vi "Initialize.vi"(8 "error in (no error)":errorcluster, 11 "VISA resource name":refnum<visa-resource-name>) -> (0 "error out":errorcluster, 3 "VISA resource name out":refnum<visa-resource-name>)   [LabVIEW 2023, in "Marlin Instrument Driver.lvlib"]
doc: "Establishes communication with the instrument and optionally performs an instrument identification query and/or an instrument reset. It also places the instrument in a default state needed for other instrument driver operations. Therefore, call this VI before calling other instrument driver VIs for this instrument. Generally, you need to call the <b>Initialize</b> VI only once at the beginning of an application."
uses:
  Marlin Instrument Driver.lvlib
panel:
  # "(c) 2021 Proper Printing.  ALL RIGHTS RESERVED."
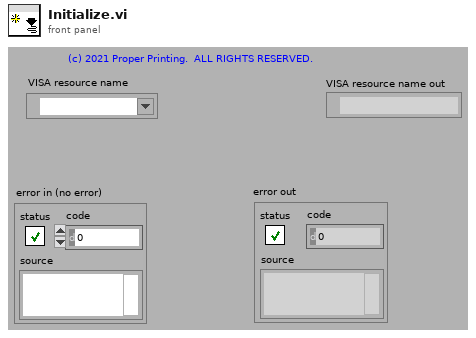
[diagram p1: front panel]
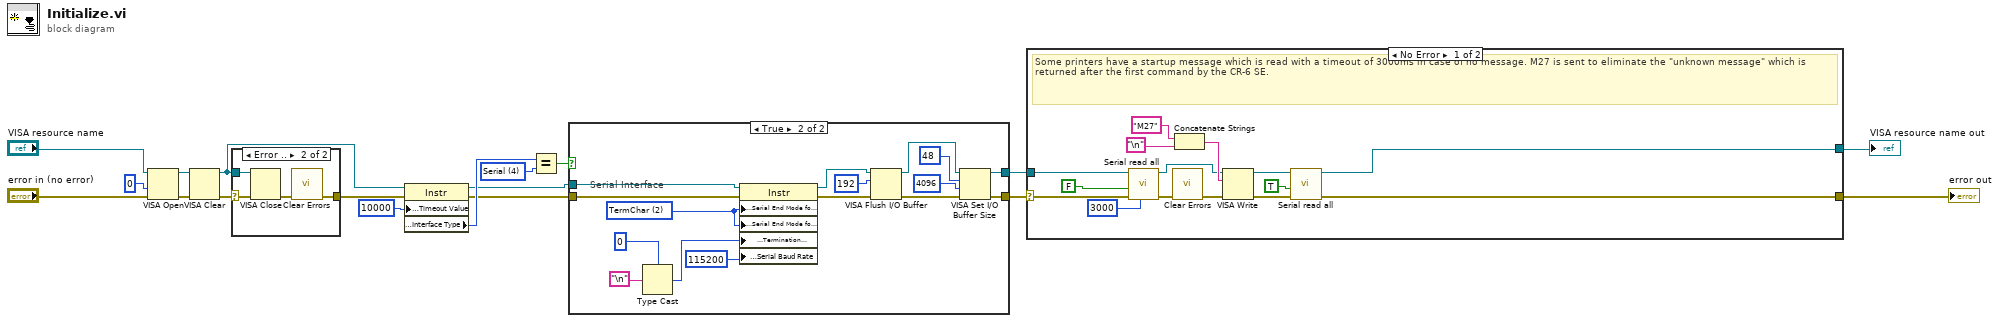
[diagram p0: block diagram]
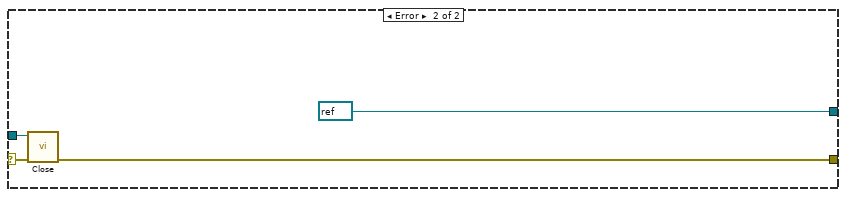
[diagram p4: hidden frame]
diagram:
  w11 = u16 4 items=["GPIB"=1, "VXI"=2, "GPIB-VXI"=3, "Serial"=4, "PXI"=5, "TCPIP"=6, "USB"=7] ("Interface Information:Interface Type")
  n1 = VISA Open(access mode=u32 0, error in (no error)="error in (no error)", VISA resource name="VISA resource name") -> (VISA resource name=w9:refnum<visa-resource-name>, error out=w8:errorcluster)  [unwired: 2 in]
  n2 = VISA Clear(VISA resource name=w9, error in (no error)=w8) -> (VISA resource name out=w1:refnum<visa-resource-name>, error out=w3:errorcluster)
  n3 = case shown="Error .." w3 {
    selector: w3 -> [w19 w22]
    tunnel: w1 -> [_ w23]
    tunnel: [w19 w20] -> w2
    frame No Error {
    }
    frame Error {
      n4 = VISA Close(VISA resource name=w23, error in (no error)=w22) -> (error out=w21:errorcluster)
      n5 = call <vilib>:"Clear Errors.vi"("error in (no error)"=w21) -> ("error out"=w20:errorcluster)  [unwired: 5 in, 1 out]
    }
  }
  n6 = property class="Instr"(reference=w1, error in=w2, "General Settings:Timeout Value"=u32 10000) -> (reference out=w14:refnum<visa-resource-name>, error out=w13:errorcluster, "Interface Information:Interface Type"=w16:u16)
  n7 = Equal?(x=w16, y=w11) -> (x = y?=w12:bool)
  n8 = case shown="True" w12 {
    tunnel: [w24 w38] -> w5
    tunnel: [w25 w35] -> w4
    tunnel: w14 -> [w24 w40]
    tunnel: w13 -> [w25 w41]
    frame False {
      # "GPIB, TCP/IP, and USB Interface"
    }
    frame True {
      w28 = u16 2 items=["None", "LastBit", "TermChar"] ("Serial Settings:Serial End Mode for Reads")
      # "Serial Interface"
      n9 = Type Cast(type=u8 0, x="\n" ("Line Feed Constant")) -> (*(type *) &x=w27:u8)
      n10 = property class="Instr"(reference=w40, error in=w41, "Serial Settings:Serial End Mode for Reads"=w28, "Serial Settings:Serial End Mode for Writes"=w28, "Message Based Settings:Termination Character"=w27, "Serial Settings:Serial Baud Rate"=u32 115200 ("Serial Settings:Baud Rate")) -> (reference out=w34:refnum<visa-resource-name>, error out=w37:errorcluster)
      n11 = VISA Flush I/O Buffer(VISA resource name=w34, mask (16)=u16 192, error in (no error)=w37) -> (VISA resource name out=w39:refnum<visa-resource-name>, error out=w36:errorcluster)
      n12 = VISA Set I/O Buffer Size(VISA resource name=w39, mask (16)=u16 48, size (4096)=u32 4096 ("size (0)"), error in (no error)=w36) -> (VISA resource name out=w38:refnum<visa-resource-name>, error out=w35:errorcluster)
    }
  }
  n13 = case shown="No Error" w4 {
    selector: w4 -> [w55 w58]
    tunnel: w5 -> [w56 w59]
    tunnel: [w43 refnum<visa-resource-name> refnum ("VISA resource name out")] -> w7
    tunnel: [w42 w60] -> w6
    frame No Error {
      # "Some printers have a startup message which is read with a timeout of 3000ms in case of no message. M27 is sent to eliminate the \"unknown message\" which is returned after the first command by the CR-6 SE."
      n14 = call "Serial read all.vi"("timeout (10000ms)"=u32 3000, "error in (no error)"=w55, "Wait for OK"=FALSE, "VISA Refnum in"=w56) -> ("error out"=w53:errorcluster, "VISA Refnum out"=w48:refnum<visa-resource-name>)  [unwired: 4 in, 2 out]
      n15 = call <vilib>:"Clear Errors.vi"("error in (no error)"=w53) -> ("error out"=w47:errorcluster)  [unwired: 5 in, 1 out]
      n16 = Concatenate Strings("M27" ("command"), "\n") -> (w50:string)
      n17 = VISA Write(VISA resource name=w48, write buffer=w50, error in (no error)=w47) -> (VISA resource name out=w44:refnum<visa-resource-name>, error out=w45:errorcluster)  [unwired: 1 out]
      n18 = call "Serial read all.vi"("error in (no error)"=w45, "Wait for OK"=TRUE, "VISA Refnum in"=w44) -> ("error out"=w42:errorcluster, "VISA Refnum out"=w43:refnum<visa-resource-name>)  [unwired: 5 in, 2 out]
    }
    frame Error {
      n19 = call "Close.vi"("error in (no error)"=w58, "VISA resource name"=w59) -> ("error out"=w60:errorcluster)  [unwired: 9 in]
    }
  }
  "VISA resource name out" <- w7
  "error out" <- w6
